vi "运维调试_CODCr.vi"() -> ()   [LabVIEW 2016, in "CODCr库.lvlib"]
uses:
  <vilib>/Utility/error.llb/DialogType.ctl
  <vilib>/Utility/miscctls.llb/LVPointTypeDef.ctl
  <vilib>/Plasmionique/MB Master/MB_Master_Serial/MB_Master_Serial.lvclass
  D:/Program Files (x86)/National Instruments/LabVIEW 2016/vi.lib/Plasmionique/MB Master/MB_Master/MB_Master.lvclass
  <vilib>/Plasmionique/MB Master/MB Master.lvlib
  <vilib>/ptbypt/NI_PtbyPt.lvlib
  <vilib>/Utility/config.llb/NI_LVConfig.lvlib
panel:
  in  "加标回收测试":bool
  in  "平行样测试":bool
  in  "定时启动":bool
  out "COM口":string
  in  "空白测试":bool
  in  "隐藏按钮":bool
  in  "写入消解温度时长":bool
  in  "保存KB值":bool
  out "source":string
  in  "标样核查":bool
  out "启动时间":timestamp format="%<%Y/%m/%d %H:%M:%S>T"
  out "主循环次数":i32
  out "status":bool
  out "启动测量模式":T1(ring)
  out "曲线斜率B":sgl format="%#_10g"
  out "曲线斜率K":sgl format="%#_10g"
  out "量程上限":sgl
  out "量程下限":sgl
  out "消解时长":u16
  out "消解温度":u16
  out "测量精度":u16
  out "测量结果":sgl
  out "标样参考值":sgl
  out "量程":u16
  out "工作状态":T1(ring)
  out "仪器时间":timestamp format="%<%X\n%x>T"
  out "关键参数区":T2
  out "状态告警区":T3
  out "测量数据区":T4 {"单位" items=["ug/L", "mg/L", "ppm", "mg/m3", "cm", "ppb", "ug/m3", "%", "nmol/mol", "umol/mol", "MPN/L", "MPN/100ml", "ng/m3", "NTU", "无量纲", "ms/cm", "us/cm", "℃", "mV", "万个/L"]}
  out "系统时间":timestamp format="%<%Y/%m/%d %H:%M:%S>T"
  in  "VISA Resource":refnum<visa-resource-name>="COM9"
  out "Registers":u16[](array[numeric])
  in  "枚举":enum16{"读取", "写入", "读取参数"}(ring)
  in  "停止":bool
  in  "校时":bool
  in  "标样校准":bool
  in  "空白校准":bool
  in  "零点核查":bool
  in  "跨度核查":bool
  in  "水样测试":bool
  in  "返回":bool
  in  "设置":bool
  # "mg/L"
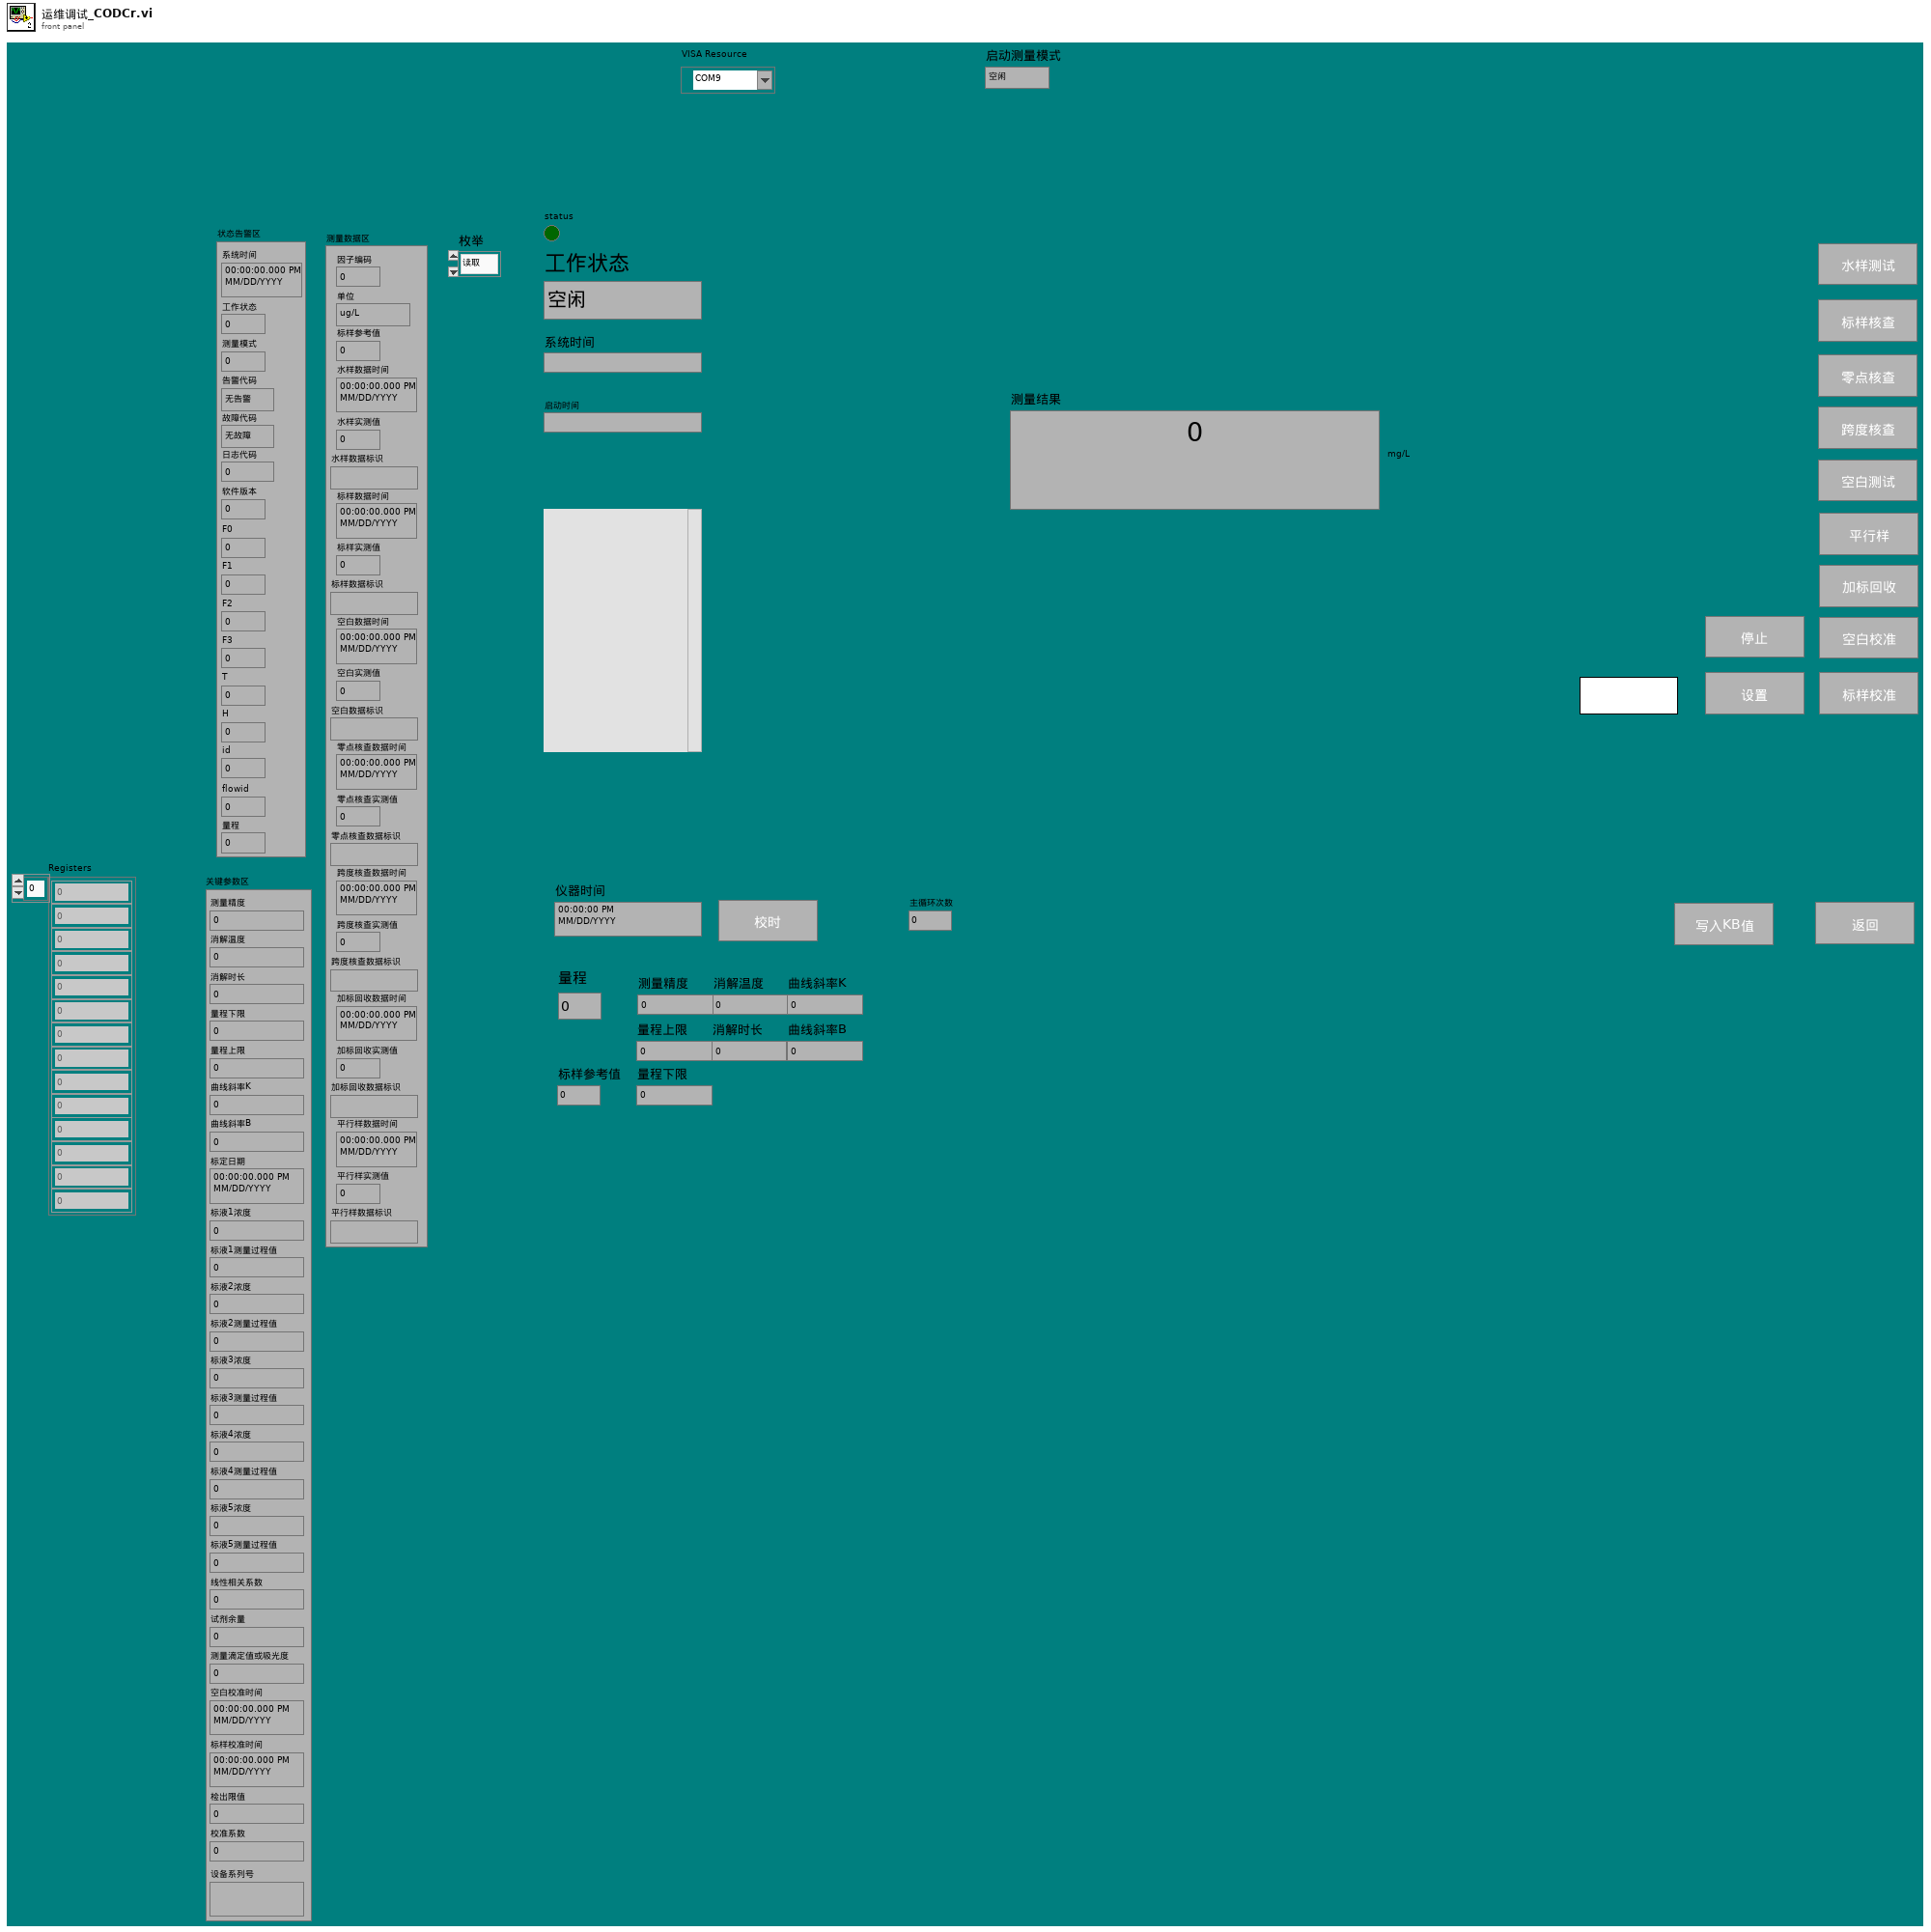
[diagram p1: front panel]
types:
  T1 = enum16{"空闲", "水样测试", "标样核查", "零点核查", "跨度核查", "空白测试", "平行样测试", "加标回收", "空白校准", "标样校准", "初始化（清洗）"}
  T2 = cluster{"测量精度":u16, "消解温度":u16, "消解时长":u16, "量程下限":sgl, "量程上限":sgl, "曲线斜率K":sgl, "曲线斜率B":sgl, "标定日期":timestamp, "标液1浓度":sgl, "标液1测量过程值":sgl, "标液2浓度":sgl, "标液2测量过程值":sgl, "标液3浓度":sgl, "标液3测量过程值":sgl, "标液4浓度":sgl, "标液4测量过程值":sgl, "标液5浓度":sgl, "标液5测量过程值":sgl, "线性相关系数":sgl, "试剂余量":u32, "测量滴定值或吸光度":sgl, "空白校准时间":timestamp, "标样校准时间":timestamp, "检出限值":sgl, "校准系数":sgl, "设备系列号":string}
  T3 = cluster{"系统时间":timestamp, "工作状态":u16, "测量模式":u16, "告警代码":enum16{"无告警", "缺试剂告警", "缺水样告警", "缺蒸馏水告警", "缺标液告警", "仪表漏液告警", "标定异常告警", "超量程告警", "加热异常", "低试剂预警", "超上限告警", "超下限告警", "仪表内部其他异常", "滴定异常告警", "电极异常告警", "量程切换告警", "参数设置告警", "PH电极电位异常", "电导率电极异常", "浊度光度异常", "溶解氧电极异常", "溶解氧光强异常", "温度异常告警", "PH异常告警", "溶解氧异常告警", "电导率异常告警", "浊度异常告警", "叶绿素异常告警", "藻密度异常告警", "蓝绿藻异常告警", "ORP异常告警", "氨氮异常告警", "清洁刷异常告警", "SD卡异常告警", "蓝牙异常告警", "Wifi异常告警", "流程异常告警"}, "故障代码":enum16{"无故障", "电机故障", "温度故障", "通讯故障", "滴定故障"}, "日志代码":u16, "软件版本":u16, "F0":sgl, "F1":sgl, "F2":sgl, "F3":sgl, "T":sgl, "H":sgl, "id":u16, "flowid":u16, "量程":u16}
  T4 = cluster{"因子编码":u32, "单位":u16, "标样参考值":sgl, "水样数据时间":timestamp, "水样实测值":sgl, "水样数据标识":string, "标样数据时间":timestamp, "标样实测值":sgl, "标样数据标识":string, "空白数据时间":timestamp, "空白实测值":sgl, "空白数据标识":string, "零点核查数据时间":timestamp, "零点核查实测值":sgl, "零点核查数据标识":string, "跨度核查数据时间":timestamp, "跨度核查实测值":sgl, "跨度核查数据标识":string, "加标回收数据时间":timestamp, "加标回收实测值":sgl, "加标回收数据标识":string, "平行样数据时间":timestamp, "平行样实测值":sgl, "平行样数据标识":string}
  T5 = cluster{"baud rate (bps)":u32, "stop bits":u16, "parity":u16, "flow control":u16, "timeout":u32, "retries":i32}
  T6 = cluster{"starting address":u16, "number of holding registers":u16}
  T7 = cluster{"测量模式":enum16{"水样测量", "标样核查", "零点核查", "跨度核查", "空白测试", "加标回收", "平行样", "校零", "校标"}}
  T8 = cluster{"仪器测试类型":enum16{"水样测试", "标样核查", "空白测试", "跨度核查"}, "周期设置类型":enum16{"定点启动", "间隔启动"}, "定时功能启用":bool, "定时间隔":dbl, "24H周期设置":bool[]}
  T9 = typedef "LVDateTimeRec.ctl" = cluster{"秒数的小数部分":dbl, "秒":i32, "分":i32, "时":i32, "日":i32, "月":i32, "年":i32, "天数（周）":i32, "天数（年）":i32, "DST":i32}
  T10 = typedef "LVPointTypeDef.ctl" = cluster{"Horizontal":i16, "Vertical":i16}
  T11 = typedef "NI_LVConfig.lvlib/Config Data RefNum.ctl" = refnum<k1>
  T12 = cluster{"运行模式":enum16{"维护模式", "常规模式", "应急模式", "质控模式"}}
  T13 = cluster{"时间标识":timestamp, "监测值":sgl, "单位":u16, "数据标识":string, "因子编码":u32, "标样参考值":sgl, "F0":sgl, "F1":sgl, "F2":sgl, "F3":sgl, "温度":sgl, "湿度":sgl, "量程标识":string}
  T14 = cluster{"时间标识":timestamp, "参数":string, "日志信息":string, "流程参数":string}
  T15 = cluster{"时间标识":timestamp, "设备":string, "日志信息":string, "流程参数":string}
  T16 = typedef "DialogType.ctl" = u16
  T17 = cluster{"系统时间":timestamp, "工作状态":enum16{"空闲", "水样测试", "标样核查", "零点核查", "跨度核查", "空白测试", "平行样测试", "加标回收", "空白校准", "标样校准", "初始化（清洗）"}, "测量模式":enum16{"待机", "连续模式", "周期模式", "定点模式", "受控模式", "手动模式"}, "告警代码":enum16{"无告警", "缺试剂告警", "缺水样告警", "缺蒸馏水告警", "缺标液告警", "仪表漏液告警", "标定异常告警", "超量程告警", "加热异常", "低试剂预警", "超上限告警", "超下限告警", "仪表内部其他异常", "滴定异常告警", "电极异常告警", "量程切换告警", "参数设置告警", "PH电极电位异常", "电导率电极异常", "浊度光度异常", "溶解氧电极异常", "溶解氧光强异常", "温度异常告警", "PH异常告警", "溶解氧异常告警", "电导率异常告警", "浊度异常告警", "叶绿素异常告警", "藻密度异常告警", "蓝绿藻异常告警", "ORP异常告警", "氨氮异常告警", "清洁刷异常告警", "SD卡异常告警", "蓝牙异常告警", "Wifi异常告警", "流程异常告警"}, "故障代码":enum16{"无故障", "电机故障", "温度故障", "通讯故障", "滴定故障"}, "日志代码":u16, "软件版本":u16, "F0":sgl, "F1":sgl, "F2":sgl, "F3":sgl, "T":sgl, "H":sgl, "id":u16, "flowid":u16, "量程":u16}
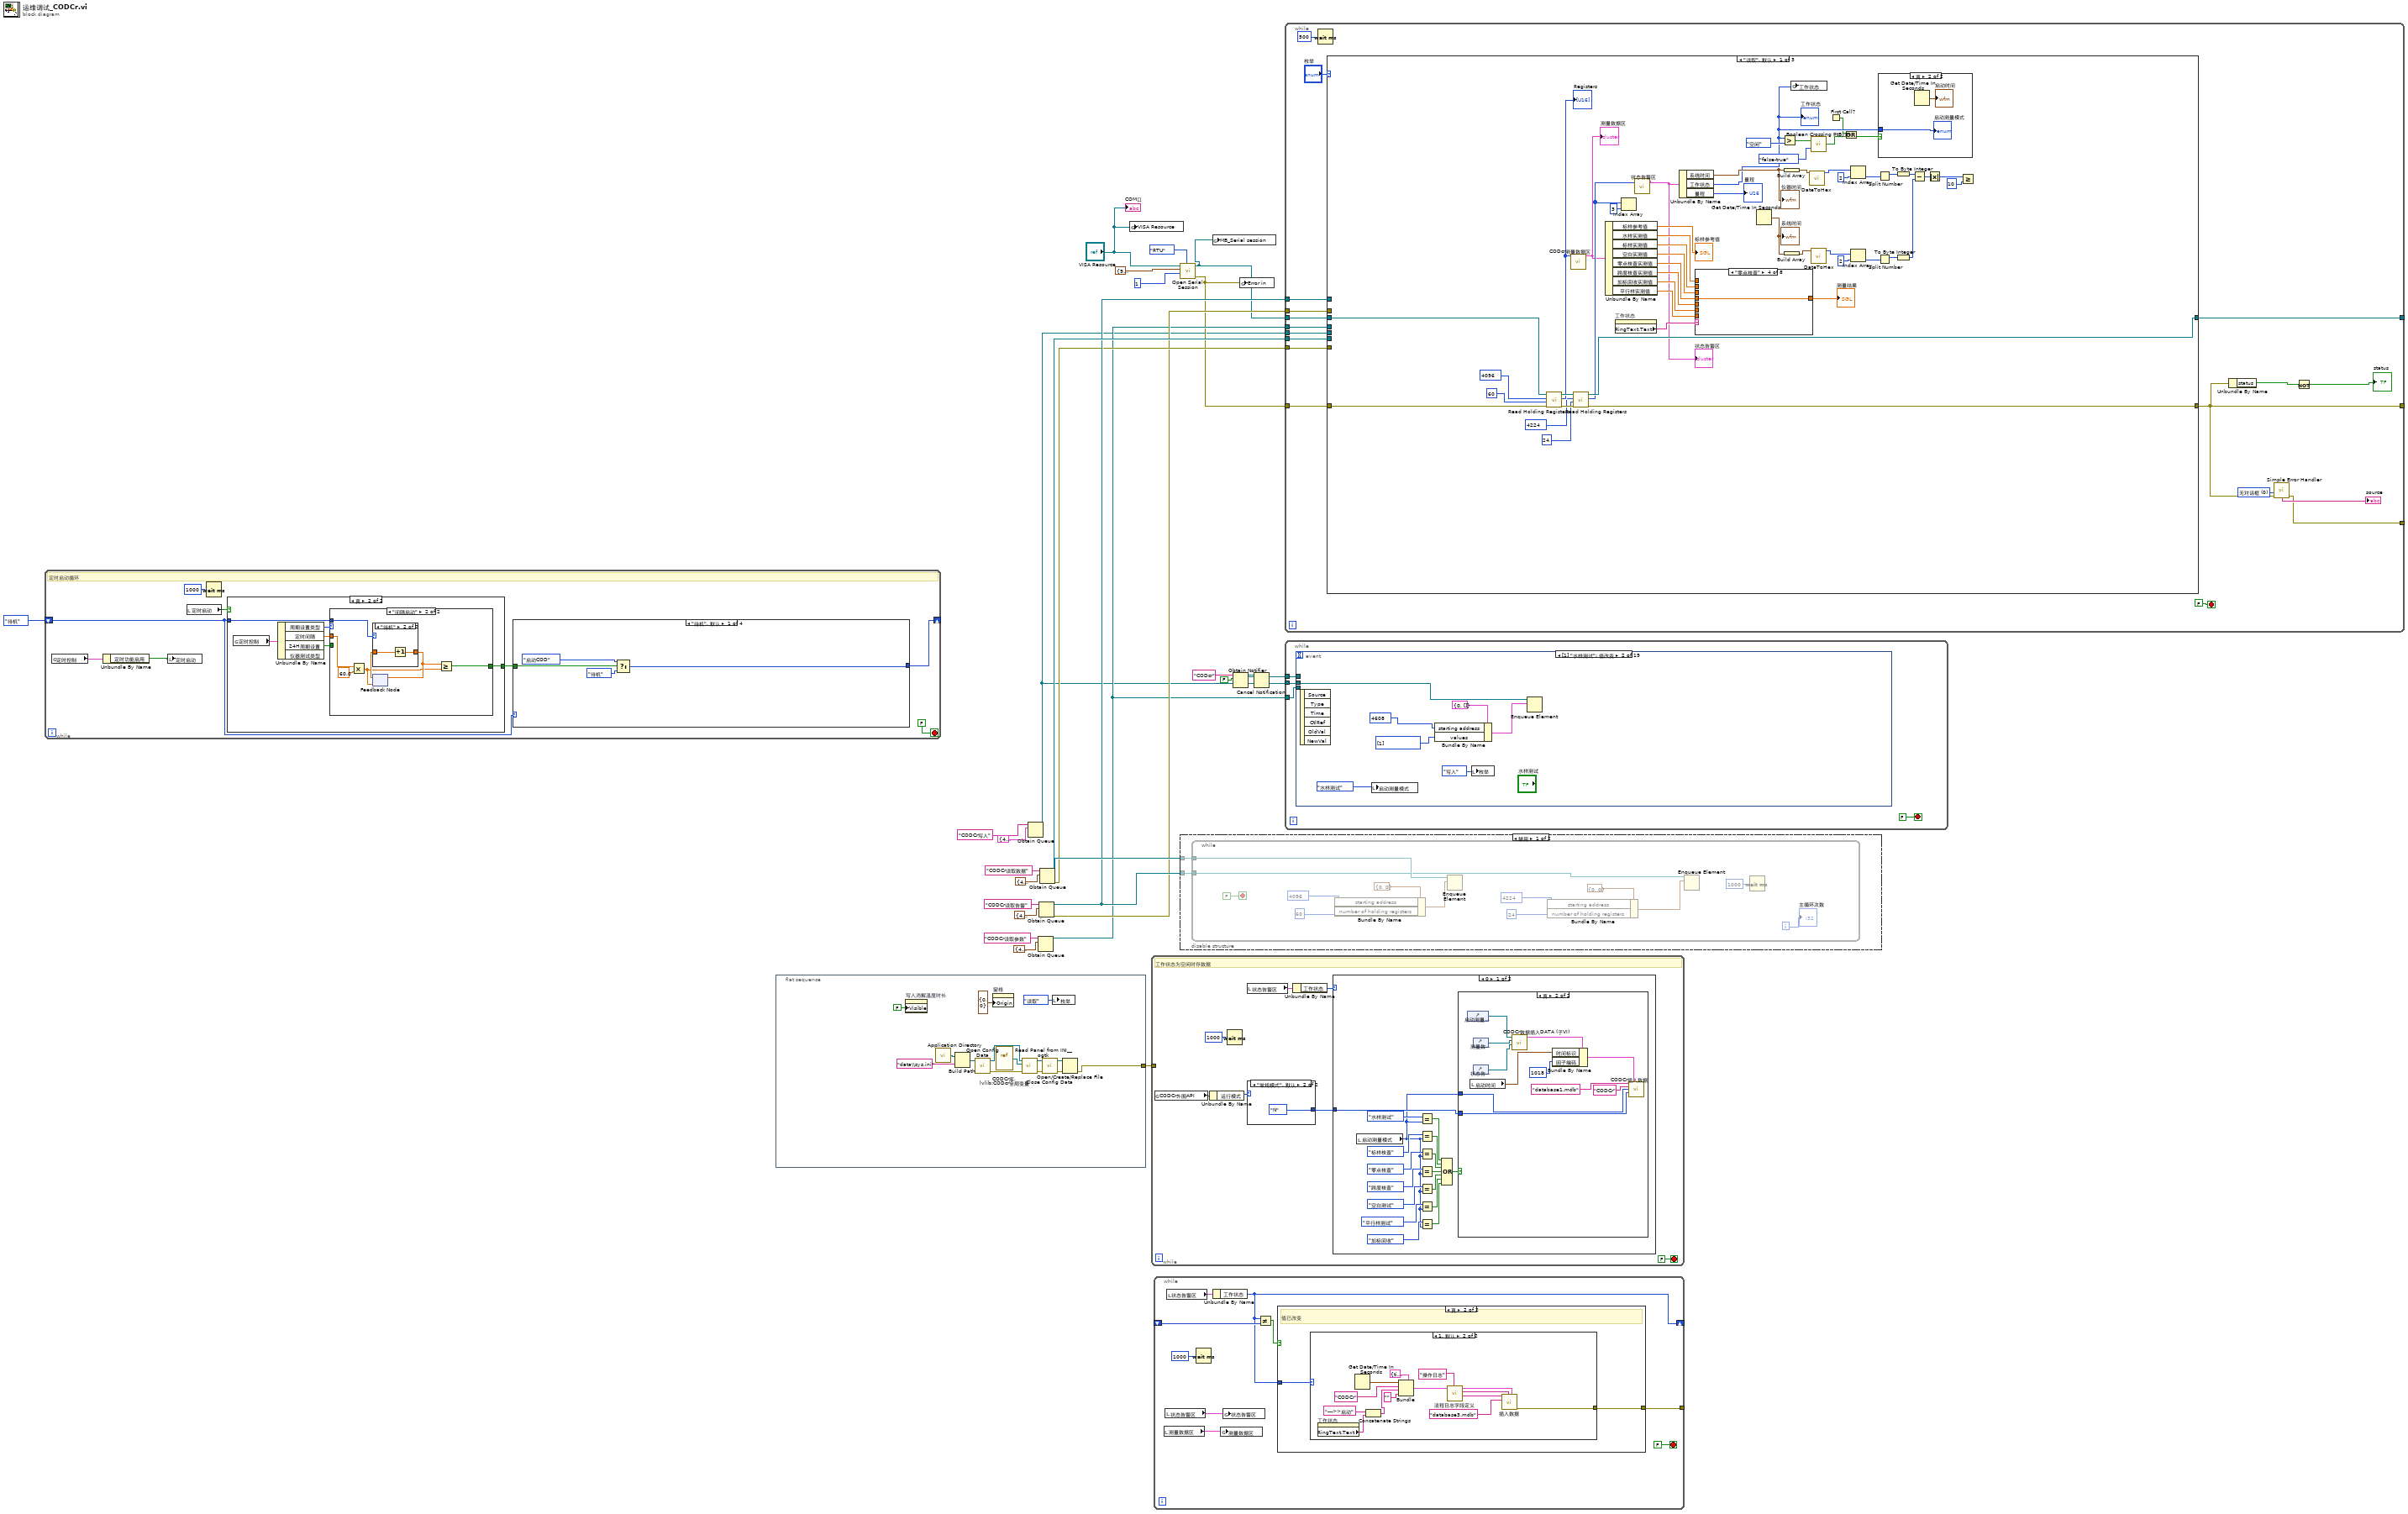
[diagram p0: block diagram]
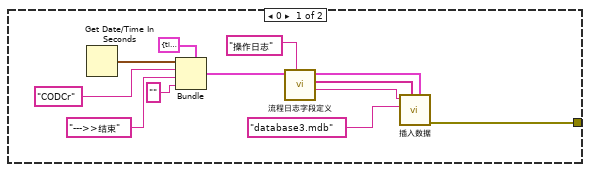
[diagram p4: hidden frame]
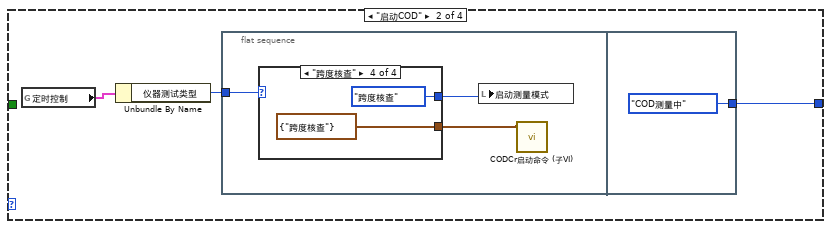
[diagram p5: hidden frame]
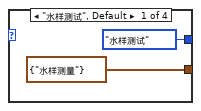
[diagram p6: hidden frame]
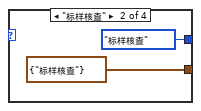
[diagram p7: hidden frame]
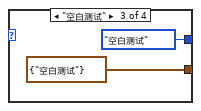
[diagram p8: hidden frame]
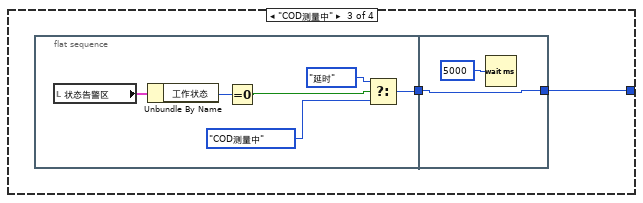
[diagram p9: hidden frame]
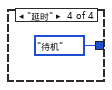
[diagram p10: hidden frame]
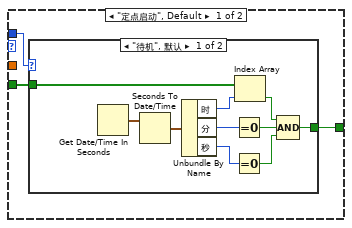
[diagram p12: hidden frame]
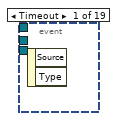
[diagram p15: hidden frame]
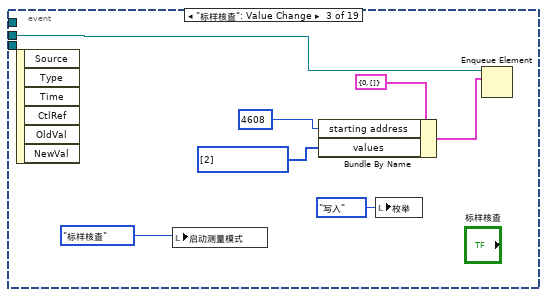
[diagram p16: hidden frame]
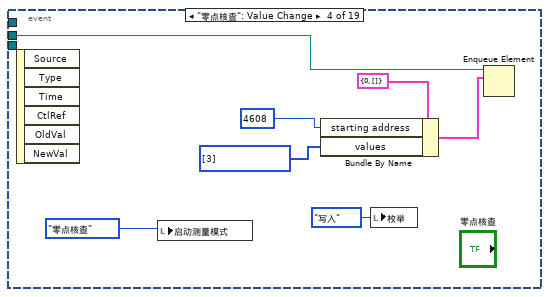
[diagram p17: hidden frame]
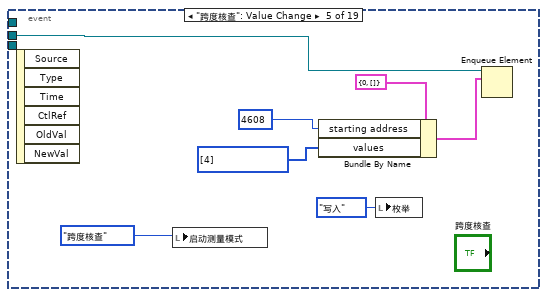
[diagram p18: hidden frame]
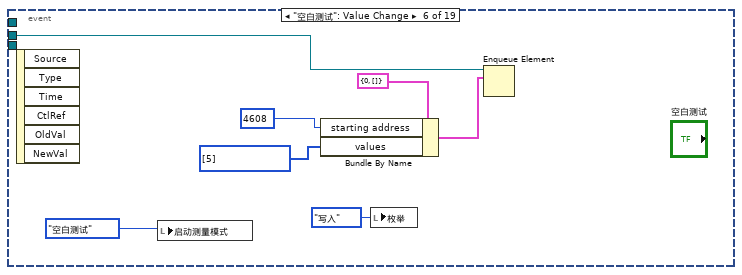
[diagram p19: hidden frame]
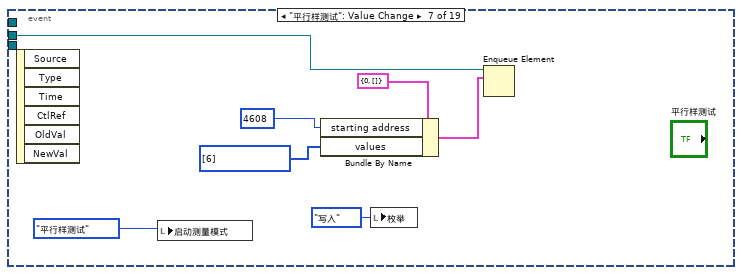
[diagram p20: hidden frame]
diagram:
  n1 = while {
    shift-right: [w32] -> _
    shift-left: enum16{"待机", "启动COD", "COD测量中", "延时"}."待机" -> [w31]
    stop <- FALSE stop-if-true
    # "定时启动循环"
    n2 = global read "CODcr全局变量.vi" "定时控制"() -> (w28:T8)
    n3 = Unbundle By Name(w28) -> ("定时功能启用"=w27:bool)
    n4 = local write "定时启动"(w27) -> ()
    n5 = local read "定时启动"() -> (w29:bool)
    n6 = Wait (ms)(milliseconds to wait=u32 1000 ("等待时间（毫秒）")) -> ()  [unwired: 1 out]
    n7 = case shown="真" w29 {
      tunnel: w31 -> [_ w67]
      tunnel: [_ w66] -> w30
      frame False {
      }
      frame True {
        n8 = global read "CODcr全局变量.vi" "定时控制"() -> (w65:T8)
        n9 = Unbundle By Name(w65) -> ("周期设置类型"=w68:enum16{"定点启动", "间隔启动"}, "定时间隔"=w69:dbl, "24H周期设置"=w70:bool[])  [unwired: 1 out]
        n10 = case shown="\"间隔启动\"" w68 {
          tunnel: w69 -> [_ w87]
          tunnel: w70 -> [w73 _]
          tunnel: w67 -> [w71 w90]
          tunnel: [w72 w85] -> w66
          frame "定点启动", Default {
            n11 = case shown="\"待机\", 默认" w71 {
              tunnel: w73 -> [w81 _]
              tunnel: [w74 _] -> w72
              frame "待机", Default {
                n12 = Get Date/Time In Seconds() -> (seconds since 1Jan1904=w83:timestamp)
                n13 = Seconds To Date/Time(time stamp (now)=w83) -> (date time rec=w82:T9)  [unwired: 1 in]
                n14 = Unbundle By Name(w82) -> ("时"=w80:i32, "分"=w78:i32, "秒"=w79:i32)
                n15 = Equal To 0?(x=w78) -> (x = 0?=w76:bool)
                n16 = Equal To 0?(x=w79) -> (x = 0?=w75:bool)
                n17 = Index Array(array=w81, index=w80) -> (element=w77:bool)
                n18 = Compound Arithmetic op=AND ("复合运算")(w77, w76, w75) -> (w74:bool)
              }
              frame "启动COD" {
              }
            }
          }
          frame "间隔启动" {
            n19 = Multiply(x=w87, y=60.0) -> (x*y=w84:dbl)
            n20 = feedback #1(w84) -> (w89:dbl)
            n21 = case shown="\"待机\"" w90 {
              tunnel: w89 -> [_ w92]
              tunnel: [_ w91] -> w88
              frame Default {
              }
              frame "待机" {
                n22 = Increment(x=w92) -> (x+1=w91:dbl)
              }
            }
            n23 = feedback-in #1(w88) -> ()
            n24 = Greater Or Equal?(x=w88, y=w84) -> (x >= y?=w85:bool)
          }
        }
      }
    }
    n25 = case shown="\"待机\", 默认" w31 {
      tunnel: [w35 w41 w55 enum16{"待机", "启动COD", "COD测量中", "延时"}."待机"] -> w32
      tunnel: w30 -> [w38 _ _ _]
      frame "待机", Default {
        n26 = Select(t=enum16{"待机", "启动COD", "COD测量中", "延时"}."启动COD", s=w38, f=enum16{"待机", "启动COD", "COD测量中", "延时"}."待机") -> (s? t:f=w35:enum16{"待机", "启动COD", "COD测量中", "延时"})
      }
      frame "启动COD" {
        n27 = global read "CODcr全局变量.vi" "定时控制"() -> (w39:T8)
        n28 = Unbundle By Name(w39) -> ("仪器测试类型"=w40:enum16{"水样测试", "标样核查", "空白测试", "跨度核查"})
        n29 = flat-sequence {
          tunnel: w40 -> [w44]
          tunnel: [enum16{"待机", "启动COD", "COD测量中", "延时"}."COD测量中"] -> w41
          frame #0 {
            n30 = case shown="\"跨度核查\"" w44 {
              tunnel: [T7 {"测量模式"=enum."水样测量"} ("启动测量模式") T7 {"测量模式"=enum."标样核查"} ("启动测量模式") T7 {"测量模式"=enum."空白测试"} ("启动测量模式") T7 {"测量模式"=enum."跨度核查"} ("启动测量模式")] -> w43
              tunnel: [T1."水样测试" ("启动测量模式") T1."标样核查" ("启动测量模式") T1."空白测试" ("启动测量模式") T1."跨度核查" ("启动测量模式")] -> w42
              frame "水样测试", Default {
              }
              frame "标样核查" {
              }
              frame "空白测试" {
              }
              frame "跨度核查" {
              }
            }
            n31 = local write "启动测量模式"(w42) -> ()
            n32 = call "CODCr启动命令 (子VI).vi"("启动测量模式"=w43) -> ()  [unwired: 11 in]
          }
          frame #1 {
          }
        }
      }
      frame "COD测量中" {
        n33 = flat-sequence {
          tunnel: [w59] -> w54
          tunnel: [w63] -> w55
          tunnel: w54 -> [w63]
          frame #0 {
            n34 = local read "状态告警区"() -> (w58:T3)
            n35 = Unbundle By Name(w58) -> ("工作状态"=w57:u16)
            n36 = Equal To 0?(x=w57) -> (x = 0?=w56:bool)
            n37 = Select(t=enum16{"待机", "启动COD", "COD测量中", "延时"}."延时", s=w56, f=enum16{"待机", "启动COD", "COD测量中", "延时"}."COD测量中") -> (s? t:f=w59:enum16{"待机", "启动COD", "COD测量中", "延时"})
          }
          frame #1 {
            n38 = Wait (ms)(milliseconds to wait=u32 5000 ("等待时间（毫秒）")) -> ()  [unwired: 1 out]
          }
        }
      }
      frame "延时" {
      }
    }
  }
  n39 = flat-sequence {
    tunnel: [w93] -> w1
    frame #0 {
      n40 = property on="写入消解温度时长" class="Bool"("Visible"=FALSE ("可见")) -> ()  [unwired: 2 in, 2 out]
      n41 = call <vilib>:"Application Directory.vi"() -> ("Application Directory"=w103:path)
      n42 = Build Path(base path=w103, name or relative path="data\\sys.ini" ("名称或相对路径")) -> (appended path=w101:path)
      n43 = call <vilib>:"Open Config Data.vi"("configuration file path"=w101) -> ("error out"=w97:errorcluster, "refnum"=w100:T11)  [unwired: 8 in, 1 out]
      n44 = property on="窗格" class="Pane"("Origin"=T10 {"Horizontal"=0, "Vertical"=0} ("原点")) -> ()  [unwired: 2 in, 2 out]
      n45 = vi-ref "CODCr库.lvlib:CODcr全局变量.vi"() -> (w99:refnum<vi>)
      n46 = call <userlib>:"Read Panel from INI__ogtk.vi"("error in (no error)"=w97, "VI ref"=w99, "refnum"=w100) -> ("error out"=w96:errorcluster, "refnum out"=w98:T11)  [unwired: 7 in]
      n47 = call <vilib>:"Close Config Data.vi"("error in (no error)"=w96, "refnum"=w98) -> ("error out"=w95:errorcluster, "file path"=w94:path)  [unwired: 8 in]
      n48 = local write "枚举"(enum16{"读取", "写入", "读取参数"}."读取" ("枚举")) -> ()
      n49 = Open/Create/Replace File(file path (use dialog)=w94, error in=w95) -> (error out=w93:errorcluster)  [unwired: 4 in, 2 out]
    }
  }
  n50 = Obtain Queue(name (unnamed)="CODCr写入" ("名称（未命名）"), element data type=cluster{"starting address":u16, "values":u16[]} {"starting address"=4096, "values"=[]}) -> (queue out=w3:refnum<queue>)  [unwired: 3 in, 2 out]
  n51 = Obtain Queue(name (unnamed)="CODCr读取参数" ("名称（未命名）"), element data type=T6 {"starting address"=4096, "number of holding registers"=100}) -> (queue out=w7:refnum<queue>)  [unwired: 3 in, 2 out]
  n52 = Obtain Queue(name (unnamed)="CODCr读取告警" ("名称（未命名）"), element data type=T6 {"starting address"=4096, "number of holding registers"=100}) -> (queue out=w16:refnum<queue>, error out=w12:errorcluster)  [unwired: 3 in, 1 out]
  n53 = Obtain Queue(name (unnamed)="CODCr读取数据" ("名称（未命名）"), element data type=T6 {"starting address"=4096, "number of holding registers"=100}) -> (queue out=w19:refnum<queue>, error out=w13:errorcluster)  [unwired: 3 in, 1 out]
  n54 = global write "CODcr全局变量.vi" "VISA Resource"("VISA Resource") -> ()
  n55 = while "While循环" {
    tunnel: w1 -> [_]
    stop <- FALSE stop-if-true
    # "工作状态为空闲时存数据"
    n56 = global read "CODCr外部API.vi" "CODCr外围API"() -> (w108:T12)
    n57 = Unbundle By Name(w108) -> ("运行模式"=w107:enum16{"维护模式", "常规模式", "应急模式", "质控模式"})
    n58 = Wait (ms)(milliseconds to wait=u32 1000 ("等待时间（毫秒）")) -> ()  [unwired: 1 out]
    n59 = local read "状态告警区"() -> (w111:T3)
    n60 = case shown="\"常规模式\", 默认" w107 {
      tunnel: [enum16{"N", "M"}."M" ("数据类型") enum16{"N", "M"}."N" ("数据类型")] -> w109
      frame "维护模式" {
      }
      frame "常规模式", Default {
      }
    }
    n61 = Unbundle By Name(w111) -> ("工作状态"=w110:u16)
    n62 = case shown="0" w110 {
      tunnel: w109 -> [w132 _]
      frame 0 {
        n63 = local read "启动测量模式"() -> (w124:T1)
        n64 = Equal?(x=T1."水样测试" ("启动测量模式"), y=w124) -> (x = y?=w123:bool)
        n65 = Equal?(x=T1."标样核查" ("启动测量模式"), y=w124) -> (x = y?=w122:bool)
        n66 = Equal?(x=T1."零点核查" ("启动测量模式"), y=w124) -> (x = y?=w121:bool)
        n67 = Equal?(x=T1."跨度核查" ("启动测量模式"), y=w124) -> (x = y?=w120:bool)
        n68 = Equal?(x=T1."空白测试" ("启动测量模式"), y=w124) -> (x = y?=w119:bool)
        n69 = Equal?(x=T1."平行样测试" ("启动测量模式"), y=w124) -> (x = y?=w118:bool)
        n70 = Equal?(x=T1."加标回收" ("启动测量模式"), y=w124) -> (x = y?=w117:bool)
        n71 = Compound Arithmetic op=OR(w123, w122, w121, w120, w119, w118, w117) -> (w116:bool)
        n72 = case shown="真" w116 {
          tunnel: w124 -> [_ w135]
          tunnel: w132 -> [_ w134]
          frame False {
          }
          frame True {
            n73 = control-ref of="启动测量模式"() -> (w142:refnum<vi>)
            n74 = local read "启动时间"() -> (w143:timestamp)
            n75 = control-ref of="测量数据区"() -> (w141:refnum<vi>)
            n76 = control-ref of="状态告警区"() -> (w140:refnum<vi>)
            n77 = call "CODCr数据插入DATA (子VI).vi"("reference 2"=w140, "reference"=w141, "Enum输入"=w142) -> ("data"=w139:T13)  [unwired: 8 in]
            n78 = Bundle By Name(cluster=w139, "时间标识"=w143, "因子编码"=u32 1018) -> (w138:T13)
            n79 = call "CODCr插入数据.vi"("database"="database1.mdb", "data"=w138, "table"="CODCr", "测量模式"=w135, "数据类型"=w134) -> ()  [unwired: 10 in, 1 out]
          }
        }
      }
      frame 1, Default {
      }
    }
  }
  n80 = while {
    shift-right: [w147] -> _
    shift-left: _ -> [w149]
    tunnel: [w146] -> _
    stop <- FALSE stop-if-true
    n81 = local read "测量数据区"() -> (w145:T4)
    n82 = local read "状态告警区"() -> (w144:T3)
    n83 = local read "状态告警区"() -> (w150:T3)
    n84 = Wait (ms)(milliseconds to wait=u32 1000 ("等待时间（毫秒）")) -> ()  [unwired: 1 out]
    n85 = Unbundle By Name(w150) -> ("工作状态"=w147:u16)
    n86 = global write "CODcr全局变量.vi" "测量数据区"(w145) -> ()
    n87 = global write "CODcr全局变量.vi" "状态告警区"(w144) -> ()
    n88 = Not Equal?(x=w147, y=w149) -> (x != y?=w148:bool)
    n89 = case shown="真" w148 {
      tunnel: w147 -> [_ w154]
      tunnel: [_ w153] -> w146
      frame False {
      }
      frame True {
        # "值已改变"
        n90 = case shown="1, 默认" w154 {
          tunnel: [w155 w170] -> w153
          frame 0 {
            n91 = Get Date/Time In Seconds() -> (seconds since 1Jan1904=w162:timestamp)
            n92 = Bundle(cluster=T14 {"时间标识"=timestamp(0 s since 1904-01-01), "参数"="", "日志信息"="", "流程参数"=""} ("data in"), "时间标识"=w162, "参数"="CODCr" ("table输入"), "日志信息"="--->>结束", "流程参数"="" ("table输入")) -> (w156:T14)
            n93 = call "流程日志字段定义.vi"("table输入"="操作日志", "data in"=w156) -> ("table输出"=w160:string, "columns"=w158:string[], "data out"=w157:T15)  [unwired: 7 in]
            n94 = call "插入数据.vi"("data"=w157, "columns"=w158, "database"="database3.mdb", "table"=w160) -> ("error out"=w155:errorcluster)  [unwired: 7 in]
          }
          frame 1, Default {
            n95 = property on="工作状态" class="Enum (严格)"() -> ("RingText.Text"=w167:string)  [unwired: 2 in, 2 out]
            n96 = Get Date/Time In Seconds() -> (seconds since 1Jan1904=w177:timestamp)
            n97 = Concatenate Strings("--->>启动" ("日志信息"), w167) -> (w168:string)
            n98 = Bundle(cluster=T14 {"时间标识"=timestamp(0 s since 1904-01-01), "参数"="", "日志信息"="", "流程参数"=""} ("data in"), "时间标识"=w177, "参数"="CODCr" ("table输入"), "日志信息"=w168, "流程参数"="" ("table输入")) -> (w176:T14)
            n99 = call "流程日志字段定义.vi"("table输入"="操作日志", "data in"=w176) -> ("table输出"=w174:string, "columns"=w172:string[], "data out"=w171:T15)  [unwired: 7 in]
            n100 = call "插入数据.vi"("data"=w171, "columns"=w172, "database"="database3.mdb", "table"=w174) -> ("error out"=w170:errorcluster)  [unwired: 7 in]
          }
        }
      }
    }
  }
  n101 = call <vilib>:"Open Serial Session.vi"("Mode (RTU)"=enum16{"RTU", "ASCII"}."RTU", "Slave ID"=u8 1, "Serial Config"=T5 {"baud rate (bps)"=9600, "stop bits"=10, "parity"=0, "flow control"=0, "timeout"=1000, "retries"=1}, "VISA Resource"="VISA Resource") -> ("Error out"=w4:errorcluster, "MB_Serial session"=w5:refnum<class "MB_Master_Serial.lvclass">)  [unwired: 6 in]
  n102 = disable-structure shown="禁用" {
    disable-tunnel: w19 -> [w182 _]
    disable-tunnel: w16 -> [w181 _]
    frame Disabled {
      n103 = while {
        tunnel: w182 -> [w193]
        tunnel: w181 -> [w184]
        i -> [w183]
        stop <- FALSE stop-if-true
        n104 = Bundle By Name(cluster=T6 {"starting address"=0, "number of holding registers"=0} ("元素"), "starting address"=u16 4096, "number of holding registers"=u16 60) -> (w191:T6)
        n105 = Enqueue Element(queue=w193, element=w191) -> ()  [unwired: 2 in, 3 out]
        n106 = Bundle By Name(cluster=T6 {"starting address"=0, "number of holding registers"=0} ("元素"), "starting address"=u16 4224, "number of holding registers"=u16 24) -> (w185:T6)
        n107 = Enqueue Element(queue=w184, element=w185) -> ()  [unwired: 2 in, 3 out]
        n108 = Wait (ms)(milliseconds to wait=u32 1000 ("等待时间（毫秒）")) -> ()  [unwired: 1 out]
        "主循环次数" <- w183
      }
    }
    frame Enabled {
    }
  }
  n109 = global write "CODcr全局变量.vi" "MB_Serial session"(w5) -> ()
  n110 = Obtain Notifier(name (unnamed)="CODcr" ("名称（未命名）"), notification data type=FALSE) -> (notifier out=w8:refnum<notifier>)  [unwired: 2 in, 2 out]
  n111 = global write "CODcr全局变量.vi" "Error in"(w4) -> ()
  n112 = Cancel Notification(0:w8) -> (8:w9:refnum<notifier>)  [unwired: 1 in, 2 out]
  n113 = while {
    tunnel: w3 -> [w210]
    tunnel: w19 -> [w209]
    tunnel: w16 -> [w208]
    tunnel: w7 -> [w207]
    tunnel: w13 -> [w205]
    tunnel: w12 -> [w204]
    tunnel: w4 -> [w203]
    tunnel: [w199] -> _
    tunnel: w5 -> [w211]
    tunnel: [w206] -> _
    tunnel: [w196] -> _
    stop <- FALSE stop-if-true
    w198 = T16 0 items=["无对话框", "确定信息", "继续或停止信息", "确定信息＋警告", "继续/停止+警告"] ("type of dialog (OK msg:1)")
    n114 = Wait (ms)(milliseconds to wait=u32 500 ("等待时间（毫秒）")) -> ()  [unwired: 1 out]
    n115 = case shown="\"读取\", 默认" "枚举" {
      tunnel: w211 -> [w263 w280 w303]
      tunnel: w203 -> [w249 w279 w302]
      tunnel: w210 -> [_ w278 _]
      tunnel: w209 -> [_ _ _]
      tunnel: w208 -> [_ _ _]
      tunnel: w207 -> [_ _ w304]
      tunnel: [w248 w274 w292] -> w199
      tunnel: [w234 w275 w293] -> w206
      tunnel: w205 -> [_ _ _]
      tunnel: w204 -> [_ _ _]
      frame "读取", Default {
        n116 = call <vilib>:"Read Holding Registers.vi"("error in (no error)"=w249, "quantity"=u16 60 ("number of holding registers"), "starting address"=u16 4096, "MB session in"=w263) -> ("error out"=w261:errorcluster, "Registers"=w225:u16[], "MB session out"=w262:refnum<class "MB_Master_Serial.lvclass">)  [unwired: 5 in]
        "Registers" <- w225
        n117 = call "CODcr测量数据区.vi"("数组"=w225) -> ("测量数据区"=w226:T4)  [unwired: 10 in]
        "测量数据区" <- w226
        n118 = call <vilib>:"Read Holding Registers.vi"("error in (no error)"=w261, "quantity"=u16 24 ("number of holding registers"), "starting address"=u16 4224, "MB session in"=w262) -> ("error out"=w248:errorcluster, "Registers"=w228:u16[], "MB session out"=w234:refnum<class "MB_Master_Serial.lvclass">)  [unwired: 5 in]
        n119 = Unbundle By Name(w226) -> ("标样参考值"=→"标样参考值":sgl, "水样实测值"=w257:sgl, "标样实测值"=w255:sgl, "空白实测值"=w252:sgl, "零点核查实测值"=w254:sgl, "跨度核查实测值"=w253:sgl, "加标回收实测值"=w250:sgl, "平行样实测值"=w251:sgl)
        n120 = property on="工作状态" class="Enum (严格)"() -> ("RingText.Text"=w258:string)  [unwired: 2 in, 2 out]
        n121 = Index Array(array=w228, index=3 ("索引")) -> ()  [unwired: 1 out]
        n122 = call "状态告警区.vi"("数组"=w228) -> ("状态告警区"=w227:T17)  [unwired: 10 in]
        "状态告警区" <- w227
        n123 = Unbundle By Name(w227) -> ("系统时间"=w235:timestamp, "工作状态"=w220:T1, "量程"=→"量程":u16)
        "仪器时间" <- w235
        "工作状态" <- w220
        n124 = case shown="\"零点核查\"" w258 {
          tunnel: w257 -> [_ w265 _ _ _ _ _ _]
          tunnel: [w264 w265 w266 w267 w268 w269 w270 w271] -> w256
          tunnel: w255 -> [_ _ w266 _ _ _ _ _]
          tunnel: w254 -> [_ _ _ w267 _ _ _ _]
          tunnel: w253 -> [_ _ _ _ w268 _ _ _]
          tunnel: w252 -> [_ _ _ _ _ w269 _ _]
          tunnel: w251 -> [_ _ _ _ _ _ w270 _]
          tunnel: w250 -> [_ _ _ _ _ _ _ w271]
          frame "空闲", Default {
            n125 = local read "测量结果"() -> (w264:sgl)
          }
          frame "水样测试" {
          }
          frame "标样核查" {
          }
          frame "零点核查" {
          }
          frame "跨度核查" {
          }
          frame "空白测试" {
          }
          frame "平行样测试" {
          }
          frame "加标回收" {
          }
        }
        "测量结果" <- w256
        n126 = Get Date/Time In Seconds() -> (seconds since 1Jan1904=w236:timestamp)
        "系统时间" <- w236
        n127 = Greater?(x=w220, y=T1."空闲") -> (0:w233:bool)
        n128 = Build Array(w235) -> (w223:timestamp[])
        n129 = Build Array(w236) -> (w224:timestamp[])
        n130 = global write "CODcr全局变量.vi" "工作状态"(w220) -> ()
        n131 = call "DateToHex.vi"("DATE"=w223) -> ("数组"=w222:u16[])  [unwired: 10 in]
        n132 = call <vilib>:"Boolean Crossing PtByPt.vi"("direction"=enum16{"either", "false-true", "true-false"}."false-true", "input"=w233) -> ("crossing"=w232:bool)  [unwired: 1 in]
        n133 = call "DateToHex.vi"("DATE"=w224) -> ("数组"=w221:u16[])  [unwired: 10 in]
        n134 = First Call?() -> (First Call?: T/F=w214:bool)
        n135 = Or(x=w214, y=w232) -> (x .or. y?=w215:bool)
        n136 = Index Array(array=w222, index=2 ("索引")) -> (element=w239:u16)
        n137 = Index Array(array=w221, index=2 ("索引")) -> (element=w238:u16)
        n138 = Split Number(x=w239) -> (hi(x)=w244:u8)  [unwired: 1 out]
        n139 = Split Number(x=w238) -> (hi(x)=w241:u8)  [unwired: 1 out]
        n140 = case shown="真" w215 {
          tunnel: w220 -> [_ w272]
          frame False {
          }
          frame True {
            n141 = Get Date/Time In Seconds() -> (seconds since 1Jan1904=→"启动时间":timestamp)
            "启动测量模式" <- w272
          }
        }
        n142 = To Byte Integer(number=w244) -> (8bit integer=w245:i8)
        n143 = To Byte Integer(number=w241) -> (8bit integer=w242:i8)
        n144 = Subtract(x=w245, y=w242) -> (x-y=w243:i8)
        n145 = Absolute Value(x=w243) -> (abs(x)=w246:i8)
        n146 = Greater Or Equal?(x=w246, y=i8 10) -> ()  [unwired: 1 out]
      }
      frame "写入" {
        n147 = flat-sequence {
          tunnel: w280 -> [w288]
          tunnel: w279 -> [w287]
          tunnel: w278 -> [w284]
          tunnel: [w286] -> w277
          tunnel: [w285] -> w276
          tunnel: w277 -> [w290]
          tunnel: w276 -> [w289]
          tunnel: [w290] -> w275
          tunnel: [w289] -> w274
          frame #0 {
            n148 = Dequeue Element(queue=w284) -> (element=w283:cluster{"starting address":u16, "values":u16[]})  [unwired: 2 in, 3 out]
            n149 = Unbundle By Name(w283) -> ("starting address"=w282:u16, "values"=w281:u16[])
            n150 = call <vilib>:"Write Multiple Registers.vi"("error in (no error)"=w287, "values"=w281, "starting address"=w282, "MB session in"=w288) -> ("error out"=w285:errorcluster, "MB session out"=w286:refnum<class "MB_Master_Serial.lvclass">)  [unwired: 6 in]
          }
          frame #1 {
            n151 = local write "枚举"(enum16{"读取", "写入", "读取参数"}."读取" ("枚举")) -> ()
          }
        }
      }
      frame "读取参数" {
        n152 = Dequeue Element(queue=w304, timeout in ms (-1)=1000 ("超时毫秒(-1)")) -> (element=w311:T6)  [unwired: 1 in, 3 out]
        n153 = local write "枚举"(enum16{"读取", "写入", "读取参数"}."读取" ("枚举")) -> ()
        n154 = Unbundle By Name(w311) -> ("starting address"=w310:u16, "number of holding registers"=w309:u16)
        n155 = call <vilib>:"Read Holding Registers.vi"("error in (no error)"=w302, "quantity"=w309, "starting address"=w310, "MB session in"=w303) -> ("error out"=w306:errorcluster, "Registers"=w308:u16[], "MB session out"=w293:refnum<class "MB_Master_Serial.lvclass">)  [unwired: 5 in]
        n156 = call "关键参数区.vi"("数组"=w308) -> ("关键参数区"=w305:T2)  [unwired: 10 in]
        "关键参数区" <- w305
        n157 = Unbundle By Name(w305) -> ("测量精度"=→"测量精度":u16, "消解温度"=→"消解温度":u16, "消解时长"=→"消解时长":u16, "量程下限"=→"量程下限":sgl, "量程上限"=→"量程上限":sgl, "曲线斜率K"=→"曲线斜率K":sgl, "曲线斜率B"=→"曲线斜率B":sgl)
        n158 = call <vilib>:"Clear Errors.vi"("error in (no error)"=w306) -> ("error out"=w292:errorcluster)  [unwired: 5 in, 1 out]
      }
    }
    n159 = Unbundle By Name(w199) -> ("status"=w202:bool)
    n160 = call <vilib>:"Simple Error Handler.vi"("type of dialog (OK msg:1)"=w198, "error in (no error)"=w199) -> ("error out"=w196:errorcluster, "message"=→"source":string)  [unwired: 3 in, 3 out]
    n161 = Not(x=w202) -> (.not. x?=→"status":bool)
  }
  n162 = while {
    tunnel: w3 -> [w314]
    tunnel: w9 -> [w313]
    tunnel: w7 -> [w312]
    stop <- FALSE stop-if-true
    n163 = event shown="[1] \"水样测试\": 值改变" {
      selector: _ -> [_ _ _ _ _ _ _ _ _ _ _ _ _ _ _ _ _ _ _]
      dyn-events: _ -> [_ _ _ _ _ _ _ _ _ _ _ _ _ _ _ _ _ _ _]
      timeout: _ -> [_ _ _ _ _ _ _ _ _ _ _ _ _ _ _ _ _ _ _]
      tunnel: w314 -> [_ w322 w325 w332 w339 w346 w353 w360 w367 w374 w382 w400 _ w422 w433 _ _ _ _]
      tunnel: w313 -> [_ _ _ _ _ _ _ _ _ _ w381 _ _ _ _ _ _ _ _]
      tunnel: w312 -> [_ _ _ _ _ _ _ _ _ _ _ _ _ _ _ w437 _ _ _]
      event Timeout {
        n164 = event-data() -> ()  [unwired: 1 in, 2 out]
      }
      event "水样测试": Value Change {
        n165 = event-data() -> ()  [unwired: 1 in, 6 out]
        n166 = local write "启动测量模式"(T1."水样测试" ("启动测量模式")) -> ()
        n167 = Bundle By Name(cluster=cluster{"starting address":u16, "values":u16[]} {"starting address"=0, "values"=[]} ("元素"), "starting address"=u16 4608, "values"=u16[] [1]) -> (w320:cluster{"starting address":u16, "values":u16[]})
        n168 = local write "枚举"(enum16{"读取", "写入", "读取参数"}."写入" ("枚举")) -> ()
        n169 = Enqueue Element(queue=w322, element=w320) -> ()  [unwired: 2 in, 3 out]
      }
      event "标样核查": Value Change {
        n170 = event-data() -> ()  [unwired: 1 in, 6 out]
        n171 = local write "启动测量模式"(T1."标样核查" ("启动测量模式")) -> ()
        n172 = Bundle By Name(cluster=cluster{"starting address":u16, "values":u16[]} {"starting address"=0, "values"=[]} ("元素"), "starting address"=u16 4608, "values"=u16[] [2]) -> (w328:cluster{"starting address":u16, "values":u16[]})
        n173 = local write "枚举"(enum16{"读取", "写入", "读取参数"}."写入" ("枚举")) -> ()
        n174 = Enqueue Element(queue=w325, element=w328) -> ()  [unwired: 2 in, 3 out]
      }
      event "零点核查": Value Change {
        n175 = event-data() -> ()  [unwired: 1 in, 6 out]
        n176 = local write "启动测量模式"(T1."零点核查" ("启动测量模式")) -> ()
        n177 = Bundle By Name(cluster=cluster{"starting address":u16, "values":u16[]} {"starting address"=0, "values"=[]} ("元素"), "starting address"=u16 4608, "values"=u16[] [3]) -> (w335:cluster{"starting address":u16, "values":u16[]})
        n178 = local write "枚举"(enum16{"读取", "写入", "读取参数"}."写入" ("枚举")) -> ()
        n179 = Enqueue Element(queue=w332, element=w335) -> ()  [unwired: 2 in, 3 out]
      }
      event "跨度核查": Value Change {
        n180 = event-data() -> ()  [unwired: 1 in, 6 out]
        n181 = local write "启动测量模式"(T1."跨度核查" ("启动测量模式")) -> ()
        n182 = Bundle By Name(cluster=cluster{"starting address":u16, "values":u16[]} {"starting address"=0, "values"=[]} ("元素"), "starting address"=u16 4608, "values"=u16[] [4]) -> (w342:cluster{"starting address":u16, "values":u16[]})
        n183 = local write "枚举"(enum16{"读取", "写入", "读取参数"}."写入" ("枚举")) -> ()
        n184 = Enqueue Element(queue=w339, element=w342) -> ()  [unwired: 2 in, 3 out]
      }
      event "空白测试": Value Change {
        n185 = event-data() -> ()  [unwired: 1 in, 6 out]
        n186 = local write "启动测量模式"(T1."空白测试" ("启动测量模式")) -> ()
        n187 = Bundle By Name(cluster=cluster{"starting address":u16, "values":u16[]} {"starting address"=0, "values"=[]} ("元素"), "starting address"=u16 4608, "values"=u16[] [5]) -> (w349:cluster{"starting address":u16, "values":u16[]})
        n188 = local write "枚举"(enum16{"读取", "写入", "读取参数"}."写入" ("枚举")) -> ()
        n189 = Enqueue Element(queue=w346, element=w349) -> ()  [unwired: 2 in, 3 out]
      }
      event "平行样测试": Value Change {
        n190 = event-data() -> ()  [unwired: 1 in, 6 out]
        n191 = local write "启动测量模式"(T1."平行样测试" ("启动测量模式")) -> ()
        n192 = Bundle By Name(cluster=cluster{"starting address":u16, "values":u16[]} {"starting address"=0, "values"=[]} ("元素"), "starting address"=u16 4608, "values"=u16[] [6]) -> (w356:cluster{"starting address":u16, "values":u16[]})
        n193 = local write "枚举"(enum16{"读取", "写入", "读取参数"}."写入" ("枚举")) -> ()
        n194 = Enqueue Element(queue=w353, element=w356) -> ()  [unwired: 2 in, 3 out]
      }
      event "加标回收测试": Value Change {
        n195 = event-data() -> ()  [unwired: 1 in, 6 out]
        n196 = local write "启动测量模式"(T1."加标回收" ("启动测量模式")) -> ()
        n197 = Bundle By Name(cluster=cluster{"starting address":u16, "values":u16[]} {"starting address"=0, "values"=[]} ("元素"), "starting address"=u16 4608, "values"=u16[] [7]) -> (w363:cluster{"starting address":u16, "values":u16[]})
        n198 = local write "枚举"(enum16{"读取", "写入", "读取参数"}."写入" ("枚举")) -> ()
        n199 = Enqueue Element(queue=w360, element=w363) -> ()  [unwired: 2 in, 3 out]
      }
      event "空白校准": Value Change {
        n200 = event-data() -> ()  [unwired: 1 in, 6 out]
        n201 = local write "启动测量模式"(T1."空白校准" ("启动测量模式")) -> ()
        n202 = Bundle By Name(cluster=cluster{"starting address":u16, "values":u16[]} {"starting address"=0, "values"=[]} ("元素"), "starting address"=u16 4608, "values"=u16[] [8]) -> (w370:cluster{"starting address":u16, "values":u16[]})
        n203 = local write "枚举"(enum16{"读取", "写入", "读取参数"}."写入" ("枚举")) -> ()
        n204 = Enqueue Element(queue=w367, element=w370) -> ()  [unwired: 2 in, 3 out]
      }
      event "标样校准": Value Change {
        n205 = event-data() -> ()  [unwired: 1 in, 6 out]
        n206 = local write "启动测量模式"(T1."标样校准" ("启动测量模式")) -> ()
        n207 = Bundle By Name(cluster=cluster{"starting address":u16, "values":u16[]} {"starting address"=0, "values"=[]} ("元素"), "starting address"=u16 4608, "values"=u16[] [9]) -> (w377:cluster{"starting address":u16, "values":u16[]})
        n208 = local write "枚举"(enum16{"读取", "写入", "读取参数"}."写入" ("枚举")) -> ()
        n209 = Enqueue Element(queue=w374, element=w377) -> ()  [unwired: 2 in, 3 out]
      }
      event "停止": Value Change {
        n210 = event-data() -> ()  [unwired: 1 in, 6 out]
        n211 = Two Button Dialog(message="确认是否停止！" ("消息")) -> (T button?=w379:bool)  [unwired: 2 in]
        n212 = case shown="真" w379 {
          tunnel: w382 -> [_ w388]
          tunnel: w381 -> [_ w386]
          frame False {
          }
          frame True {
            n213 = Cancel Notification(0:w386) -> (8:w385:refnum<notifier>)  [unwired: 1 in, 2 out]
            n214 = local write "启动测量模式"(T1."空闲" ("启动测量模式")) -> ()
            n215 = Send Notification(notification=TRUE ("通知"), notifier=w385) -> ()  [unwired: 1 in, 2 out]
            n216 = Bundle By Name(cluster=cluster{"starting address":u16, "values":u16[]} {"starting address"=0, "values"=[]} ("元素"), "starting address"=u16 4608, "values"=u16[] [12]) -> (w391:cluster{"starting address":u16, "values":u16[]})
            n217 = local write "枚举"(enum16{"读取", "写入", "读取参数"}."写入" ("枚举")) -> ()
            n218 = Enqueue Element(queue=w388, element=w391) -> ()  [unwired: 2 in, 3 out]
          }
        }
      }
      event "保存KB值": Value Change {
        n219 = event-data() -> ()  [unwired: 1 in, 6 out]
        n220 = local read "曲线斜率B"() -> (w395:sgl)
        n221 = local read "曲线斜率K"() -> (w396:sgl)
        n222 = Build Array(w396, w395) -> (w394:sgl[])
        n223 = call "FloatToHex.vi"("浮点数"=w394) -> ("DCBA整形输出"=w393:u16[])  [unwired: 10 in]
        n224 = Bundle By Name(cluster=cluster{"starting address":u16, "values":u16[]} {"starting address"=0, "values"=[]} ("元素"), "starting address"=u16 4263, "values"=w393) -> (w398:cluster{"starting address":u16, "values":u16[]})
        n225 = Enqueue Element(queue=w400, element=w398) -> ()  [unwired: 2 in, 3 out]
        n226 = local write "枚举"(enum16{"读取", "写入", "读取参数"}."写入" ("枚举")) -> ()
      }
      event "定时启动": Value Change {
        n227 = event-data() -> ()  [unwired: 1 in, 6 out]
        n228 = flat-sequence {
          frame #0 {
            n229 = global read "CODcr全局变量.vi" "定时控制"() -> (w403:T8)
            n230 = call "周期设置.vi"("定时控制参数输入"=w403) -> ("定时控制参数输出"=w402:T8)  [unwired: 10 in]
            n231 = global write "CODcr全局变量.vi" "定时控制"(w402) -> ()
          }
          frame #1 {
            n232 = call <vilib>:"Application Directory.vi"() -> ("Application Directory"=w417:path)
            n233 = Build Path(base path=w417, name or relative path="data\\sys.ini" ("名称或相对路径")) -> (appended path=w415:path)
            n234 = call <vilib>:"Open Config Data.vi"("configuration file path"=w415) -> ("error out"=w411:errorcluster, "refnum"=w414:T11)  [unwired: 8 in, 1 out]
            n235 = vi-ref "CODCr库.lvlib:CODcr全局变量.vi"() -> (w413:refnum<vi>)
            n236 = call <userlib>:"Write Panel to INI__ogtk.vi"("error in (no error)"=w411, "VI ref"=w413, "refnum"=w414) -> ("error out"=w410:errorcluster, "refnum out"=w412:T11)  [unwired: 7 in]
            n237 = call <vilib>:"Close Config Data.vi"("error in (no error)"=w410, "refnum"=w412) -> ("error out"=w405:errorcluster, "file path"=w404:path)  [unwired: 8 in]
            n238 = Open/Create/Replace File(file path (use dialog)=w404, error in=w405) -> (refnum out=w408:refnum<file>, error out=w409:errorcluster)  [unwired: 4 in, 1 out]
            n239 = Flush File(refnum=w408, error in=w409) -> (refnum out=w407:refnum<file>, error out=w406:errorcluster)
            n240 = Close File(refnum=w407, error in=w406) -> ()  [unwired: 2 out]
          }
        }
      }
      event "写入消解温度时长": Value Change {
        n241 = event-data() -> ()  [unwired: 1 in, 6 out]
        n242 = local read "消解时长"() -> (w420:u16)
        n243 = local read "消解温度"() -> (w421:u16)
        n244 = Build Array(w421, w420) -> (w419:u16[])
        n245 = call "WordToHex.vi"("WORD"=w419) -> ("数组"=w418:u16[])  [unwired: 10 in]
        n246 = Bundle By Name(cluster=cluster{"starting address":u16, "values":u16[]} {"starting address"=0, "values"=[]} ("元素"), "starting address"=u16 4257, "values"=w418) -> (w424:cluster{"starting address":u16, "values":u16[]})
        n247 = Enqueue Element(queue=w422, element=w424) -> ()  [unwired: 2 in, 3 out]
      }
      event "校时": Value Change {
        n248 = event-data() -> ()  [unwired: 1 in, 6 out]
        n249 = Get Date/Time In Seconds() -> (seconds since 1Jan1904=w432:timestamp)
        n250 = Build Array(w432) -> (w427:timestamp[])
        n251 = call "DateToHex.vi"("DATE"=w427) -> ("数组"=w426:u16[])  [unwired: 10 in]
        n252 = Insert Into Array(array=u16[] [13] ("values"), index=1 ("索引"), new element=w426) -> (w429:u16[])
        n253 = local write "枚举"(enum16{"读取", "写入", "读取参数"}."写入" ("枚举")) -> ()
        n254 = Bundle By Name(cluster=cluster{"starting address":u16, "values":u16[]} {"starting address"=0, "values"=[]} ("元素"), "starting address"=u16 4608, "values"=w429) -> (w435:cluster{"starting address":u16, "values":u16[]})
        n255 = Enqueue Element(queue=w433, element=w435) -> ()  [unwired: 2 in, 3 out]
      }
      event "设置": Value Change {
        n256 = event-data() -> ()  [unwired: 1 in, 6 out]
        n257 = property on="窗格" class="Pane"("Origin"=T10 {"Horizontal"=0, "Vertical"=728} ("原点")) -> ()  [unwired: 2 in, 2 out]
        n258 = flat-sequence {
          tunnel: w437 -> [w439]
          frame #0 {
            n259 = Bundle By Name(cluster=T6 {"starting address"=0, "number of holding registers"=0} ("元素"), "starting address"=u16 4256, "number of holding registers"=u16 19) -> (w443:T6)
            n260 = Enqueue Element(queue=w439, element=w443) -> ()  [unwired: 2 in, 3 out]
          }
          frame #1 {
            n261 = local write "枚举"(enum16{"读取", "写入", "读取参数"}."读取参数" ("枚举")) -> ()
          }
        }
      }
      event "返回": Value Change {
        n262 = event-data() -> ()  [unwired: 1 in, 6 out]
        n263 = property on="窗格" class="Pane"("Origin"=T10 {"Horizontal"=0, "Vertical"=0} ("原点")) -> ()  [unwired: 2 in, 2 out]
        n264 = property on="写入消解温度时长" class="Bool"("Visible"=FALSE ("可见")) -> ()  [unwired: 2 in, 2 out]
      }
      event "曲线斜率K", "曲线斜率B", "消解温度", "消解时长": Mouse Down {
        n265 = event-data() -> ("CtlRef"=w449:refnum<vi>)  [unwired: 1 in, 7 out]
        n266 = property class="DigNum"(reference=w449) -> (reference out=w450:refnum<vi>, "Value"=w448:variant)  [unwired: 1 in, 1 out]
        n267 = Variant To Data(Variant=w448) -> (data=w447:sgl)  [unwired: 2 in, 1 out]
        n268 = call "CODCR数字键盘.vi"("OldNumber"=w447) -> ("NewNumber"=w451:sgl)
        n269 = property class="DigNum"(reference=w450, "Value"=w451) -> ()  [unwired: 1 in, 2 out]
      }
      event "隐藏按钮": Value Change {
        n270 = event-data() -> ()  [unwired: 1 in, 6 out]
        n271 = property on="写入消解温度时长" class="Bool"("Visible"=TRUE ("可见")) -> ()  [unwired: 2 in, 2 out]
      }
    }
  }
  "COM口" <- "VISA Resource"
